vi "util_transition_criteria.vi"(8 "error in (no error)":errorcluster, 9 "next_index":i32=-1, 10 "data":variant, 11 "recipe_data":variant) -> (0 "error out":errorcluster)   [LabVIEW 2015, in "lv-recipe-machine.lvlib"]
uses:
  lv-recipe-machine.lvlib
  _controls/transition.ctl
  _controls/change.ctl
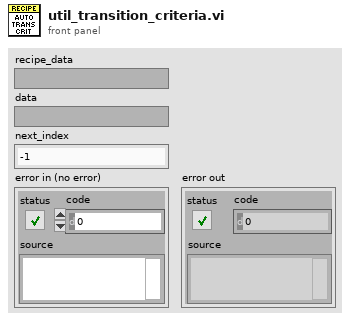
[diagram p1: front panel]
types:
  T1 = cluster{"change_in_event":refnum<user-event>, "transition_queue":refnum<queue>}
  T2 = cluster{"change_in_event":bool, "transition_queue":bool}
  T3 = typedef "lv-recipe-machine.lvlib/references.ctl" = cluster{"semaphore":T4, "input_queue":refnum<queue>, "output_queue":refnum<queue>, "transition_queue":refnum<queue>, "data_dvr":refnum<data-value>, "stop_notifier":refnum<notifier>, "change_in_event":refnum<user-event>, "change_out_event":refnum<user-event>, "status_event":refnum<user-event>}
  T4 = typedef "Semaphore RefNum" = refnum<k1>
  T5 = typedef "lv-recipe-machine.lvlib/transition.ctl" = cluster{"next_index":i32, "data":variant, "recipe_data":variant, "error":errorcluster}
  T6 = typedef "lv-recipe-machine.lvlib/change.ctl" = cluster{"data":variant}
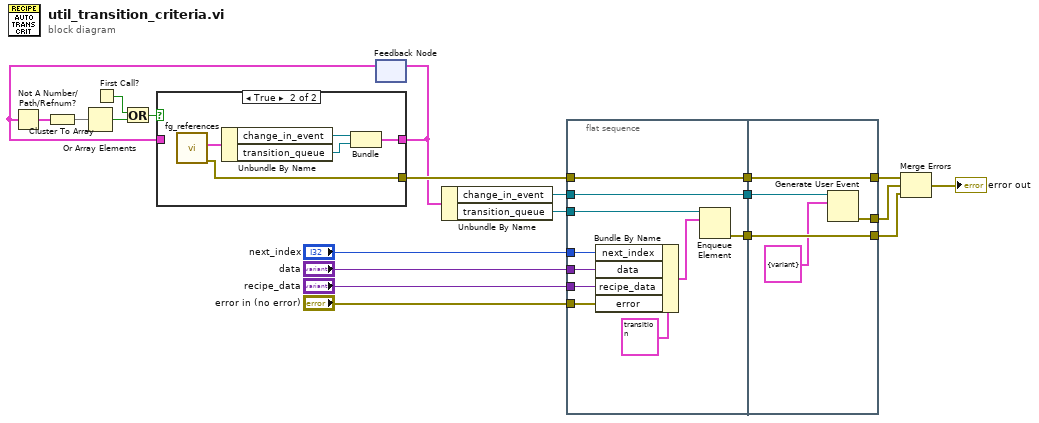
[diagram p0: block diagram]
diagram:
  n1 = First Call?() -> (First Call?: T/F=w10:bool)
  n2 = feedback #1() -> (w9:T1)  [unwired: 1 in]
  n3 = Not A Number/Path/Refnum?(number/path/refnum=w9) -> (NaN/Path/Refnum?=w11:T2)
  n4 = Cluster To Array(cluster=w11) -> (array=w7:bool[])
  n5 = Or Array Elements(Boolean array=w7) -> (logical OR=w6:bool)
  n6 = Or(x=w10, y=w6) -> (x .or. y?=w8:bool)
  n7 = case shown="True" w8 {
    tunnel: [_ w27] -> w21
    tunnel: [w22 w24] -> w5
    tunnel: w9 -> [w22 _]
    frame False {
    }
    frame True {
      n8 = call "fg_references.vi"() -> ("error out"=w27:errorcluster, "references out"=w26:T3)  [unwired: 10 in]
      n9 = Unbundle By Name(w26) -> ("change_in_event"=w25:refnum<user-event>, "transition_queue"=w23:refnum<queue>)
      n10 = Bundle("change_in_event"=w25, "transition_queue"=w23) -> (w24:T1)  [unwired: 1 in]
    }
  }
  n11 = feedback-in #1(w5) -> ()
  n12 = Unbundle By Name(w5) -> ("change_in_event"=w3:refnum<user-event>, "transition_queue"=w4:refnum<queue>)
  n13 = flat-sequence {
    tunnel: w3 -> [w36]
    tunnel: w4 -> [w37]
    tunnel: [w36] -> w18
    tunnel: "next_index" -> [w33]
    tunnel: "data" -> [w32]
    tunnel: "recipe_data" -> [w31]
    tunnel: "error in (no error)" -> [w30]
    tunnel: [w29] -> w13
    tunnel: w21 -> [w28]
    tunnel: [w28] -> w2
    tunnel: [w41] -> w20
    tunnel: w18 -> [w40]
    tunnel: w13 -> [w42]
    tunnel: [w42] -> w12
    tunnel: w2 -> [w38]
    tunnel: [w38] -> w1
    frame #0 {
      n14 = Bundle By Name(cluster=T5 {"next_index"=0, "data"=variant, "recipe_data"=variant, "error"={"status"=FALSE, "code"=0, "source"=""}} ("transition"), "next_index"=w33, "data"=w32, "recipe_data"=w31, "error"=w30) -> (w34:T5)
      n15 = Enqueue Element(queue=w37, element=w34) -> (error out=w29:errorcluster)  [unwired: 2 in, 2 out]
    }
    frame #1 {
      n16 = Generate User Event(user event=w40, event data cluster=T6 {"data"=variant} ("event data")) -> (error out=w41:errorcluster)  [unwired: 2 in, 1 out]
    }
  }
  n17 = Merge Errors(w1, w20, w12) -> (→"error out":errorcluster)
